vi "全局变量.vi"() -> ()   [LabVIEW 2018]
panel:
  in  "已开盖次数":dbl
  out "关盖缓冲异常":bool
  out "开盖缓冲异常":bool
  in  "zds4":dbl
  in  "zds3":dbl
  in  "zds2":dbl
  in  "zds1":dbl
  in  "zds8":dbl
  in  "zds7":dbl
  in  "zds6":dbl
  in  "zds5":dbl
  in  "sds4":dbl
  in  "sds3":dbl
  in  "sds2":dbl
  in  "sds1":dbl
  in  "sds8":dbl
  in  "sds7":dbl
  in  "sds6":dbl
  in  "sds5":dbl
  in  "Switch":dbl
  in  "Switch1":dbl
  in  "Switch2":dbl
  in  "tsyajin":dbl
  in  "tsguangai":dbl
  in  "tsjiesuo":dbl
  in  "tssuoding":dbl
  in  "tskaigai":dbl
  in  "tssongkai":dbl
  in  "tskaishi8":dbl
  in  "tskaishi7":dbl
  in  "tskaishi6":dbl
  in  "tskaishi5":dbl
  in  "tskaishi4":dbl
  in  "tskaishi3":dbl
  in  "tskaishi2":dbl
  in  "tskaishi1":dbl
  out "sd压紧异常":bool
  out "sd关盖异常":bool
  out "sd解锁异常":bool
  out "sd锁定异常":bool
  out "sd开盖异常":bool
  out "sd松开异常":bool
  out "zd压紧异常":bool
  out "zd关盖异常":bool
  out "zd解锁异常":bool
  out "zd锁定异常":bool
  out "zd开盖异常":bool
  out "zd松开异常":bool
  in  "qiehuan":dbl
  in  "tiaoshimoshi":dbl
  in  "c4":dbl
  in  "c3":dbl
  in  "c2":dbl
  in  "c1":dbl
  in  "c8":dbl
  in  "c7":dbl
  in  "c6":dbl
  in  "c5":dbl
  in  "qidongsd":dbl
  in  "qidongzd":dbl
  in  "passt":dbl
  in  "s4":dbl
  in  "s3":dbl
  in  "s2":dbl
  in  "s1":dbl
  in  "s8":dbl
  in  "s7":dbl
  in  "s6":dbl
  in  "s5":dbl
  in  "yajintm":dbl
  in  "guangaitm":dbl
  in  "jiesuotm":dbl
  in  "suodingtm":dbl
  in  "kaigaitm":dbl
  in  "songkaitm":dbl
  in  "guanzhiling1":dbl
  in  "kaizhiling1":dbl
  in  "yajin":dbl
  in  "guangai":dbl
  in  "jiesuo":dbl
  in  "suoding":dbl
  in  "kaigai":dbl
  in  "songkai":dbl
  in  "tuichu":dbl
  in  "guanzhi":dbl
  in  "kaizhi":dbl
  in  "time2":dbl
  in  "time1":dbl
  in  "pass1":dbl
  in  "pass":dbl
  in  "zidong":dbl
  in  "t6":dbl
  in  "t5":dbl
  in  "t4":dbl
  in  "t3":dbl
  in  "t2":dbl
  in  "t1":dbl
  in  "guan7":dbl
  in  "ya7":dbl
  in  "kai7":dbl
  in  "song7":dbl
  in  "guan6":dbl
  in  "ya6":dbl
  in  "kai6":dbl
  in  "song6":dbl
  in  "guan5":dbl
  in  "ya5":dbl
  in  "kai5":dbl
  in  "song5":dbl
  in  "guan4":dbl
  in  "ya4":dbl
  in  "kai4":dbl
  in  "song4":dbl
  in  "guan3":dbl
  in  "ya3":dbl
  in  "kai3":dbl
  in  "song3":dbl
  in  "guan2":dbl
  in  "ya2":dbl
  in  "kai2":dbl
  in  "song2":dbl
  in  "guan1":dbl
  in  "ya1":dbl
  in  "kai1":dbl
  in  "song1":dbl
  in  "kaishi8":dbl
  in  "kaishi7":dbl
  in  "kaishi6":dbl
  in  "kaishi5":dbl
  in  "kaishi4":dbl
  in  "kaishi3":dbl
  in  "kaishi2":dbl
  in  "kaishi1":dbl
  out "退出系统":bool
  in  "Resetdog1":dbl
  out "关盖指令2":bool
  out "关盖指令1":bool
  out "关盖换向阀":bool
  out "压紧换向阀":bool
  out "开盖指令2":bool
  out "开盖指令1":bool
  out "开盖换向阀":bool
  out "松开换向阀":bool
  in  "guan0":dbl
  in  "ya0":dbl
  in  "kai0":dbl
  in  "song0":dbl
  in  "energy_stop":dbl
  in  "shengguang":dbl
  in  "recheck":dbl
  in  "kaigaicishu":dbl
  in  "kaishi":dbl
  out "cuowu":bool[](array[boolean])
  in  "ScopeData":dbl[][](array[numeric])
  in  "ScopeData_Unpack":dbl[][](array[numeric])
  in  "Time":dbl[](array[numeric])
  out "ScopeFinish":bool
  in  "数据储存":bool
  out "关盖缓冲":bool
  out "error":bool
  out "check_ok":bool
  out "关盖到位2":bool
  out "关盖到位1":bool
  out "压紧到位":bool
  out "锁定到位":bool
  out "开盖缓冲":bool
  out "开盖到位2":bool
  out "开盖到位1":bool
  out "松开到位":bool
  out "解锁到位":bool
  in  "Resetdog":dbl
  in  "Reset":dbl
  in  "jieshu":dbl
  in  "start":dbl
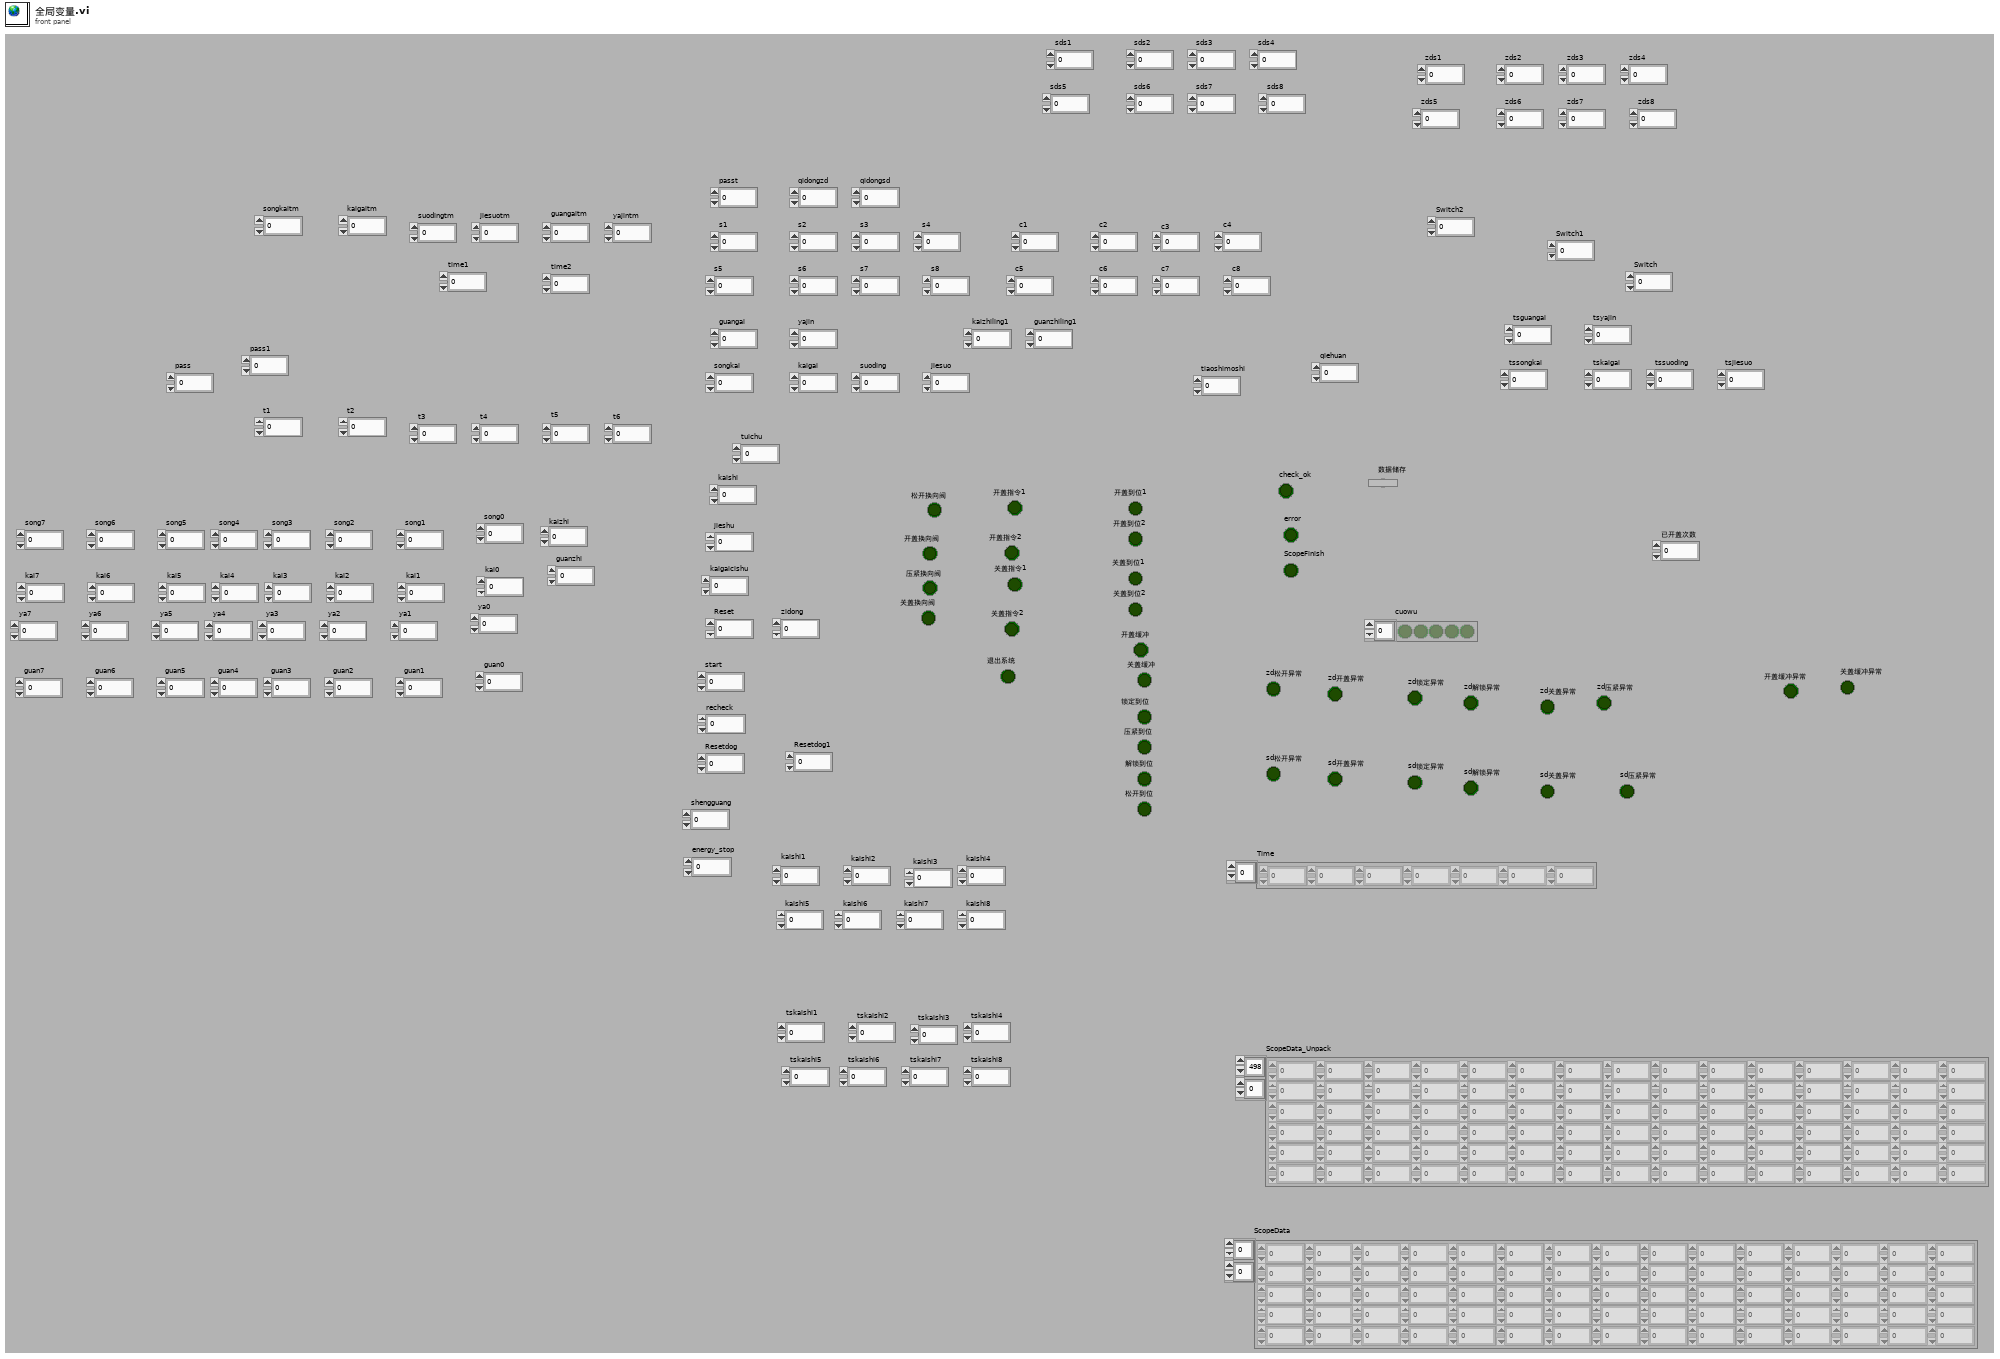
[diagram p1: front panel]
diagram:
